vi "Handler.vi"() -> ()   [LabVIEW 2018]
uses:
  QueueNames.ctl
  <vilib>/NI/AMC/Read Termination Message.vi
  <vilib>/NI/AMC/Create Single Message.vi
  <vilib>/NI/AMC/Update Message Routing Info.vi
  <vilib>/NI/AMC/Globals.vi
  <vilib>/NI/AMC/Send Message.vi
  <vilib>/NI/AMC/AMC.lvlib
panel:
  in  "PXI Musashi":string[](array[string])=["DIO:", "6509", "Counter:", "6733_1", "Slow AO:", "6704", "Fast AO:", "6733_1", "6733_2"]
  in  "PXI Positron":string[](array[string])=["DIO:", "6509", "Counter:", "6733_1", "Slow AO:", "6723", "Fast AO:", "6733_1", "6733_2", "6733_3"]
  in  "PXI Cusp":string[](array[string])=["DIO:", "6509", "Counter:", "6733_1", "Slow AO:", "6723", "Fast AO:", "6733_1", "6733_2"]
  in  "System":u16(ring)=1 items=["Cusp", "Positron", "Musashi"]
  in  "Target Port":u16=6378
  in  "Host process":string="GUI"
  in  "Host port":u16=6674
  out "Local Error":errorcluster
  out "Closed OK?":string[](array[string])=["RT Loop VI Closed", "ParameterChange VI Closed"]
  in  "stop":bool
  # "auto-rampdown for slow AO?"
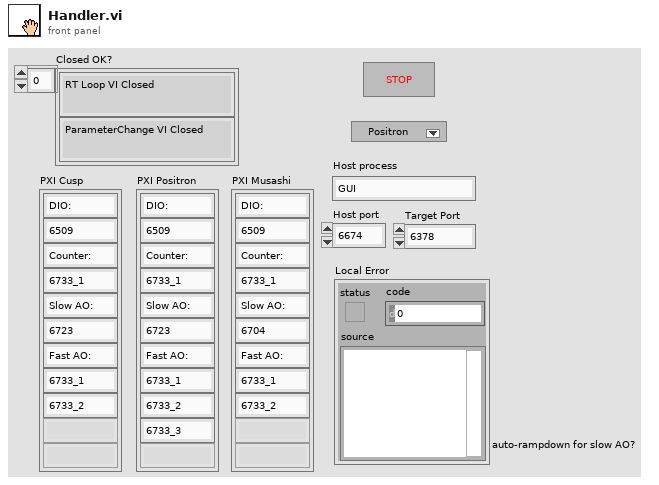
[diagram p1: front panel]
types:
  T1 = typedef "QueueNames.ctl" = enum32{"Handler", "RT Loop", "Slow AO"}
  T2 = typedef "AMC.lvlib/Message Queue.ctl" = refnum<queue>
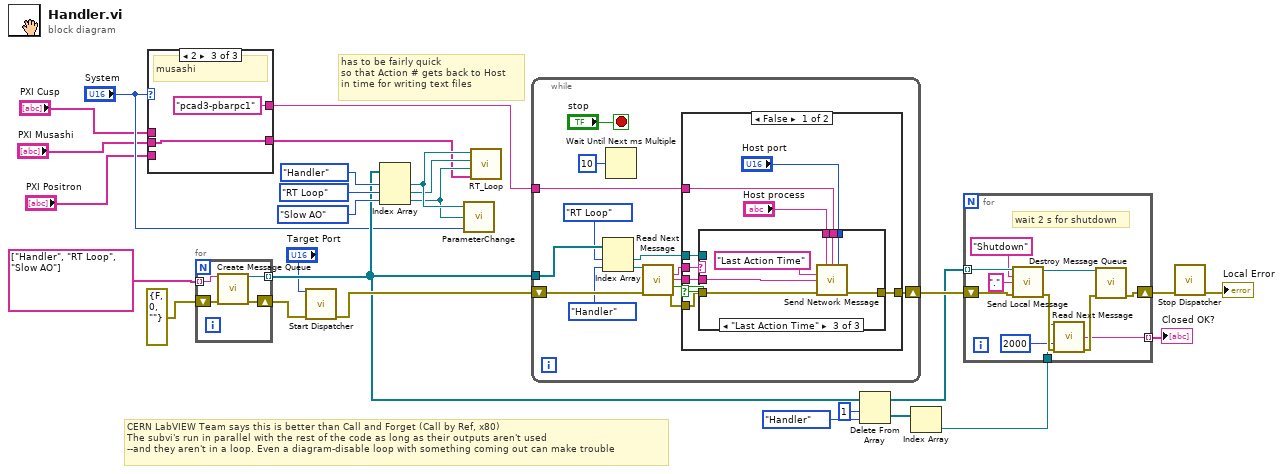
[diagram p0: block diagram]
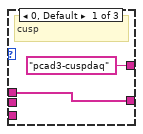
[diagram p2: hidden frame]
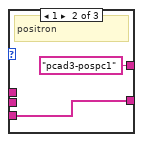
[diagram p3: hidden frame]
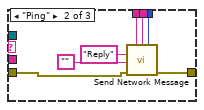
[diagram p5: hidden frame]
diagram:
  # "CERN LabVIEW Team says this is better than Call and Forget (Call by Ref, x80)\nThe subvi's run in parallel with the rest of the code as long as their outputs aren't used\n--and they aren't in a loop. Even a diagram-disable loop with something coming out can make trouble"
  # "has to be fairly quick \nso that Action # gets back to Host \nin time for writing text files"
  n1 = case shown="2" "System" {
    tunnel: ["pcad3-cuspdaq" ("Host IP") "pcad3-pospc1" ("Host IP") "pcad3-pbarpc1" ("Host IP")] -> w6
    tunnel: [w28 w30 w32] -> w4
    tunnel: "PXI Positron" -> [_ w30 _]
    tunnel: "PXI Cusp" -> [w28 _ _]
    tunnel: "PXI Musashi" -> [_ _ w32]
    frame 0, Default {
      # "cusp"
    }
    frame 1 {
      # "positron"
    }
    frame 2 {
      # "musashi"
    }
  }
  n2 = for {
    tunnel: string[] ["Handler", "RT Loop", "Slow AO"] ("Strings []") -> [w36] mode=indexing
    tunnel: [w35] -> w11 mode=indexing
    shift-right: [w34] -> w10
    shift-left: errorcluster {"status"=FALSE, "code"=0, "source"=""} ("error out") -> [w37]
    n3 = call <vilib>:"Create Message Queue.vi"("message queue name"=w36, "error in"=w37) -> ("message queue out"=w35:T2, "error out"=w34:errorcluster)  [unwired: 12 in]
  }
  n4 = call <vilib>:"Start Dispatcher.vi"("UDP port (0)"="Target Port", "error in"=w10) -> ("error out"=w18:errorcluster)  [unwired: 11 in, 2 out]
  n5 = Index Array(array=w11, index #1=QueueNames."Handler" ("Queue Name Refs"), index #2=QueueNames."RT Loop" ("Queue Name Refs"), index #3=QueueNames."Slow AO" ("Queue Name Refs")) -> (element #1=w14:T2, element #2=w13:T2, element #3=w12:T2)
  n6 = call "ParameterChange.vi"("System"="System", "Slow AO Qname"=w12, "Handler Qname"=w14) -> ()  [unwired: 2 in]
  n7 = call "RT_Loop.vi"("PXI card names"=w4, "Param Qname"=w12, "RT Loop Qname"=w13, "Handler Qname"=w14) -> ()
  n8 = while {
    shift-right: [w41] -> w26
    shift-left: w18 -> [w49]
    tunnel: w11 -> [w50]
    tunnel: w6 -> [w38]
    stop <- "stop" stop-if-true
    n9 = Index Array(array=w50, index #1=QueueNames."RT Loop" ("Queue Name Refs"), index #2=QueueNames."Handler" ("Queue Name Refs")) -> (element #1=w39:T2, element #2=w45:T2)
    n10 = Wait Until Next ms Multiple(millisecond multiple=u32 10) -> ()  [unwired: 1 out]
    n11 = call <vilib>:"Read Next Message.vi"("message queue in"=w45, "error in"=w49) -> ("message name"=w46:string, "message value"=w44:string, "timed out?"=w47:bool, "error out"=w42:errorcluster)  [unwired: 6 in, 4 out]
    n12 = case shown="False" w47 {
      tunnel: w46 -> [w59 _]
      tunnel: w44 -> [w58 _]
      tunnel: w42 -> [w56 w75]
      tunnel: [w55 w75] -> w41
      tunnel: w39 -> [w57 _]
      tunnel: w38 -> [w52 _]
      frame False {
        n13 = case shown="\"Last Action Time\"" w59 {
          tunnel: w58 -> [_ _ w73]
          tunnel: w57 -> [_ _ _]
          tunnel: w56 -> [w60 w62 w72]
          tunnel: [w60 w61 w74] -> w55
          tunnel: "Host port" -> [_ w67 w70]
          tunnel: "Host process" -> [_ w65 w69]
          tunnel: w52 -> [_ w66 w68]
          frame Default {
          }
          frame "Ping" {
            n14 = call <vilib>:"Send Network Message.vi"("receiver process"=w65, "receiver host"=w66, "receiver port (0)"=w67, "message name"="Reply", "message value"="", "error in"=w62) -> ("error out"=w61:errorcluster)  [unwired: 7 in, 2 out]
          }
          frame "Last Action Time" {
            n15 = call <vilib>:"Send Network Message.vi"("receiver process"=w69, "receiver host"=w68, "receiver port (0)"=w70, "message name"="Last Action Time", "message value"=w73, "error in"=w72) -> ("error out"=w74:errorcluster)  [unwired: 7 in, 2 out]
          }
        }
      }
      frame True {
        # "timed out"
      }
    }
  }
  n16 = Delete From Array(array=w11, length=1, index=QueueNames."Handler" ("Queue Name Refs")) -> (deleted portion=w21:T2[], array with subset deleted=w22:T2[])
  n17 = Index Array(array=w21) -> (element=w20:T2)  [unwired: 1 in]
  n18 = for {
    shift-right: [w86] -> w27
    shift-left: w26 -> [w85]
    tunnel: w22 -> [w84] mode=indexing
    tunnel: [w79] -> w25 mode=indexing
    tunnel: w20 -> [w78]
    # "wait 2 s for shutdown"
    n19 = call <vilib>:"Send Local Message.vi"("message queue in"=w84, "message name"="Shutdown", "message value"=".", "error in"=w85) -> ("message queue out"=w77:T2, "error out"=w82:errorcluster)  [unwired: 9 in, 1 out]
    n20 = call <vilib>:"Read Next Message.vi"("message queue in"=w78, "timeout (1 ms)"=2000, "error in"=w82) -> ("message value"=w79:string, "error out"=w81:errorcluster)  [unwired: 5 in, 6 out]
    n21 = call <vilib>:"Destroy Message Queue.vi"("message queue in"=w77, "error in"=w81) -> ("error out"=w86:errorcluster)  [unwired: 11 in, 2 out]
  }
  "Closed OK?" <- w25
  n22 = call <vilib>:"Stop Dispatcher.vi"("error in"=w27) -> ("error out"=→"Local Error":errorcluster)  [unwired: 14 in]
